vi "Synchros Final.vi"() -> ()   [LabVIEW 2014]
panel:
  out "x >= y?":bool
  in  "Tab Control":T1(tab)
  out "?":i32
  in  "?":dbl(knob) scale=0.0..360.0
  out "?":dbl(knob) scale=0.0..360.0
  out "?":dbl(knob) scale=0.0..360.0
  out "?":dbl(knob) scale=0.0..360.0
  out "?":i32
  in  "?":enum16{"S1 and S2", "S2 and S3", "S1 and S3"}(ring)
  out "?":dbl format="%#_4g"
  out "?":bool
  out "?":bool
  in  "STOP":bool
  in  "STOP  .":bool
  out "1":string[][](table)
  in  "?":dbl(slide)=29.292929292929294 scale=0.0..100.0
  out "?":dbl
  out "?":dbl(knob) scale=0.0..360.0
  out "?":dbl(knob) scale=0.0..360.0
  out "?":dbl(knob) scale=0.0..360.0
  out "?":dbl
  out "?":dbl
  in  "?":enum16{"S1 and S2", "S2 and S3", "S1 and S3"}(ring)
  out "?":dbl format="%#_4g"
  out "?":dbl(knob) scale=0.0..360.0
  out "Position Vs Stator Voltage":cluster{"Y":dbl[], "Y":dbl[]}[](graph)
  out "?":bool
  out "?":bool
  # "Manipal Institute of Technology  \n        Dept of Instrumentation and Control Engineering\n                                 V Sem (Instrumentation Lab)"
  # "VIRTUAL LABS"
  # "VIRTUAL LABS"
  # "Characteristics of Synchros\nAim:\nTo measure the Stator output voltage with respect to rotor position and plot the graph. \nApparatus required:\n1.\tSynchro Transmitter / Receiver (PEC 03) Trainer kit.\n2.\tPatch chords\n\nInstructions:\n\tConnect Digital Voltmeter across any two Stator output of Synchro transmitter.\n1.\tConnect Synchro transmitter stator outputs to corresponding Stator terminals of Synchro receiver.\n2.\tPower 'ON'  all ON/OFF Switches\n3.\tVerify the Stator output voltage of 0V at 0 degree, if it is not make 0V at 0 degree to adjust the pointer of both transmitter and Receiver.\n4.\tAdjust the transmitter rotor position Step by Step.\n5.\tNote down the output voltage for various rotor position in table 1.\n6.\tNote down the rotor position of transmitter and receiver in table 2.\n7.\tRepeat the Same procedure for other pair of Synchro transmitter coils.\n\n\nMotor graph:"
  # "EXPERIMENT NO.1"
  # "Angular Displacement\n(in deg)"
  # "Angular Displacement\n(in deg)"
  # "Reciever"
  # "Transmitter"
  # "S1"
  # "S2"
  # "S3"
  # "S1"
  # "S2"
  # "S3"
  # "Select coils for Voltage  \n    Measurement"
  # "Voltage (V)"
  # "Angular Displacement\n(in deg)"
  # "Angular Displacement\n(in deg)"
  # "Animation Speed"
  # "Reciever"
  # "Transmitter"
  # "S1"
  # "S2"
  # "S3"
  # "S1"
  # "S2"
  # "S3"
  # "Select coils for Voltage  \n    Measurement"
  # "Voltage (V)"
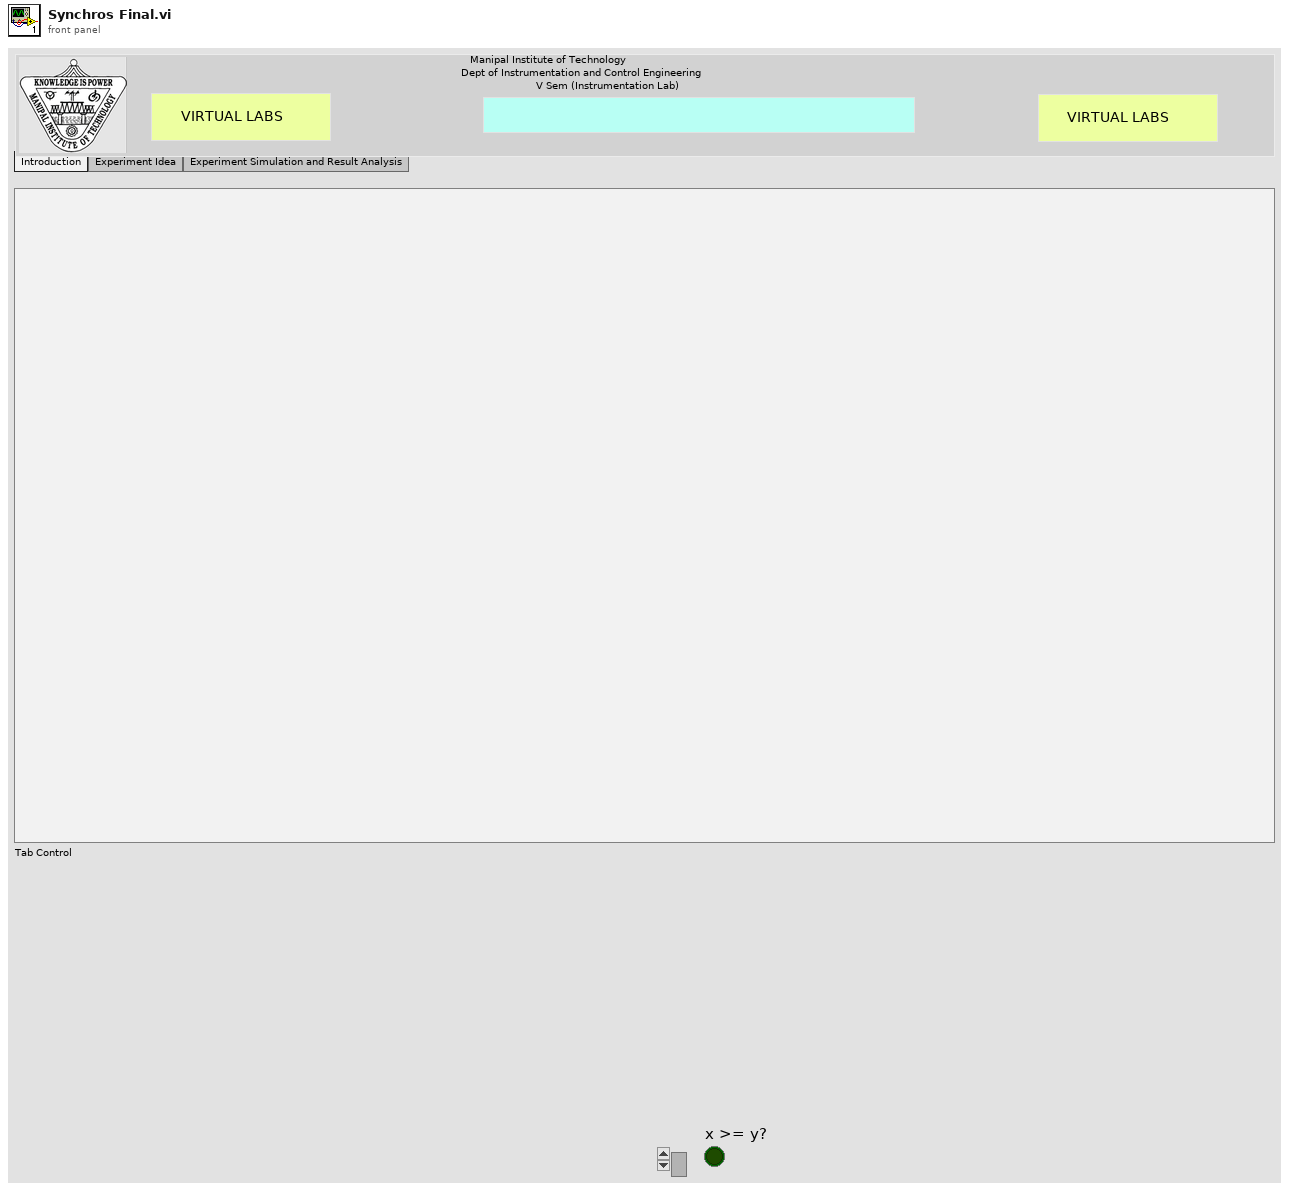
[diagram p1: front panel]
types:
  T1 = enum32{"Introduction", "Experiment Idea", "Experiment Simulation and Result Analysis"}
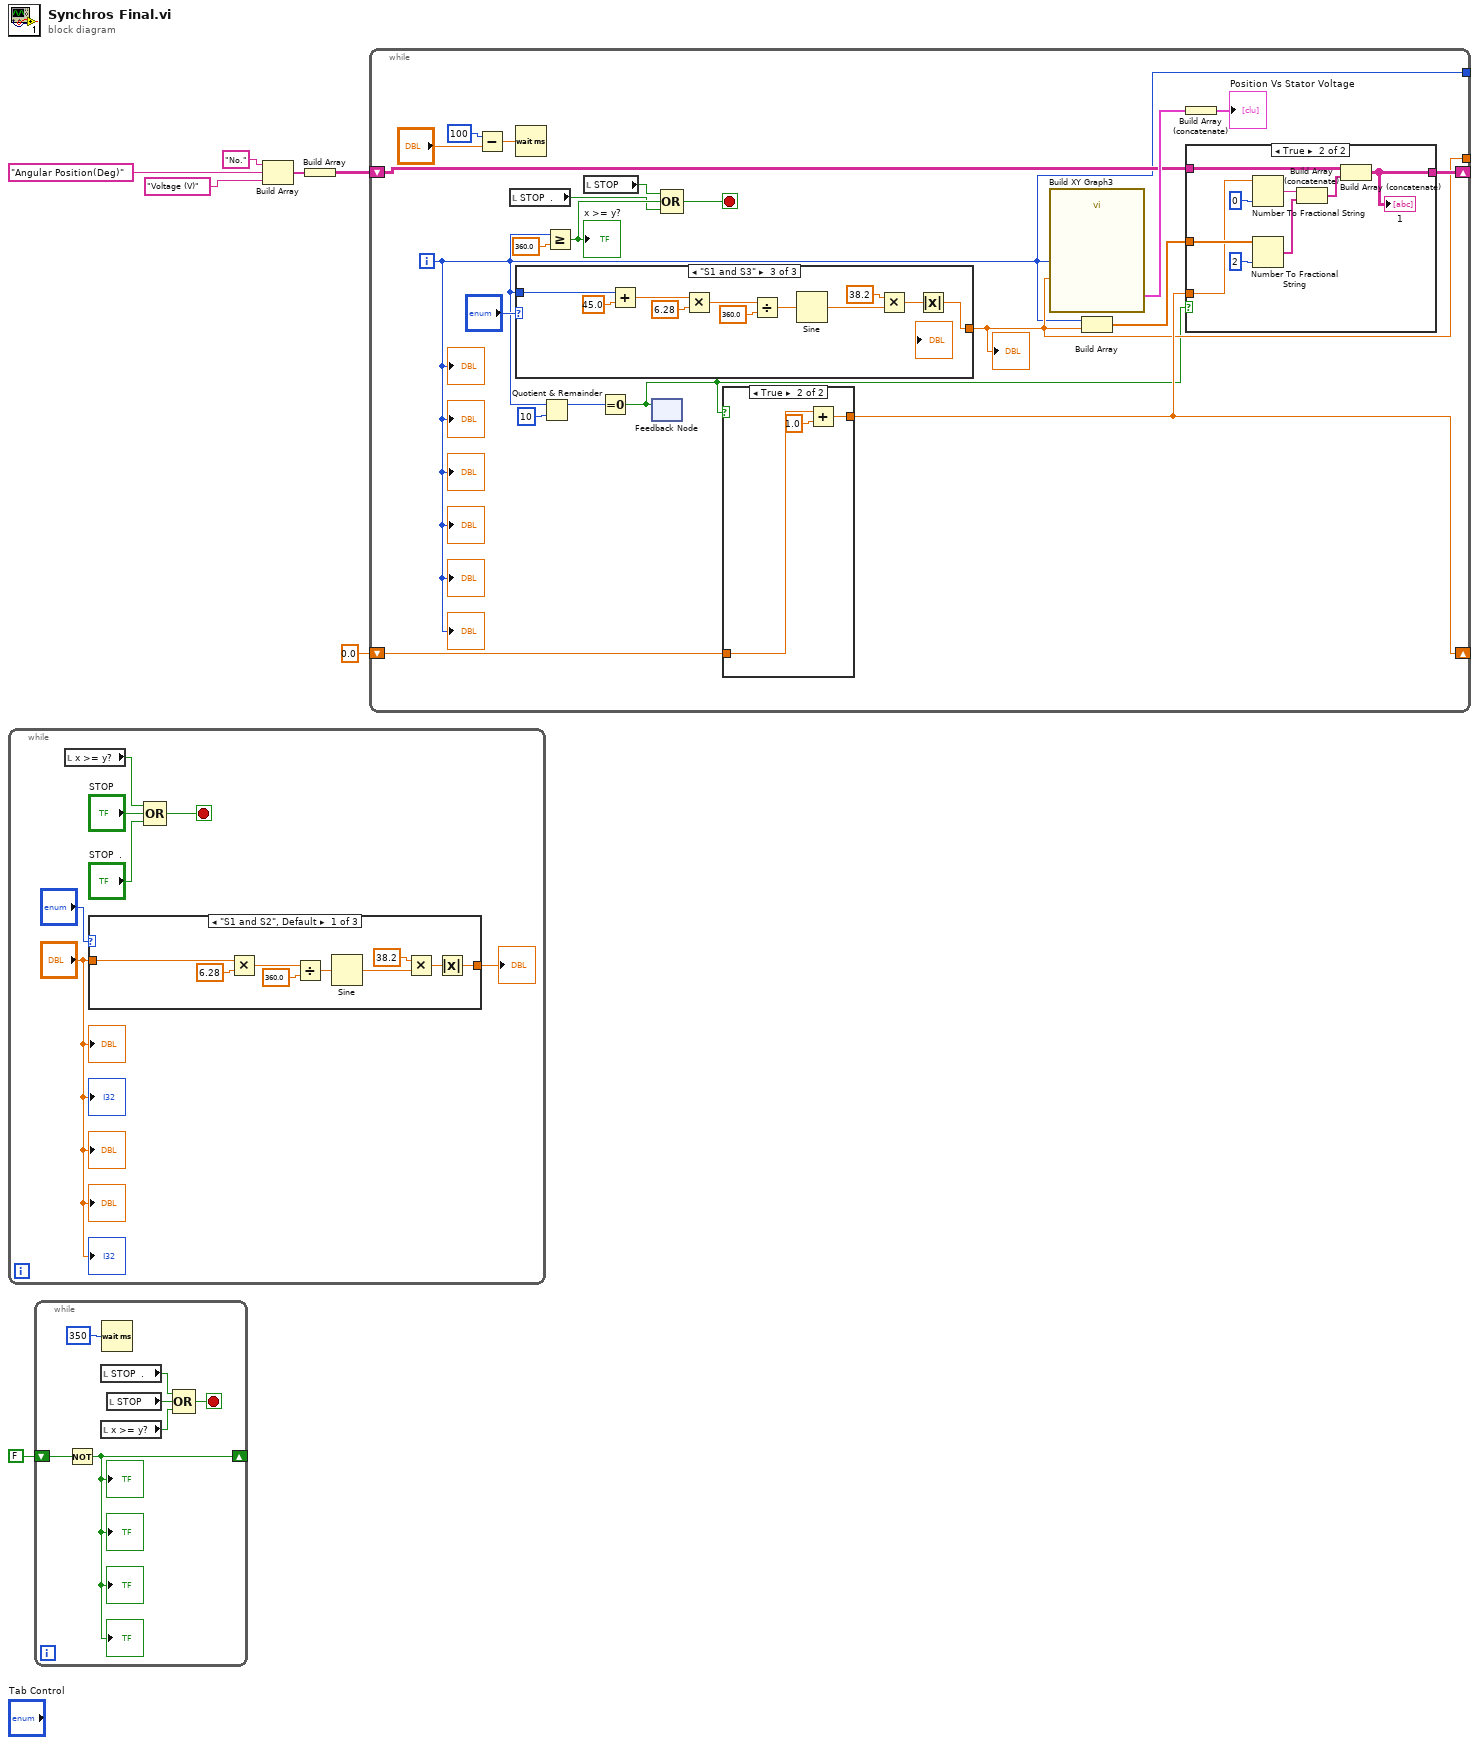
[diagram p0: block diagram]
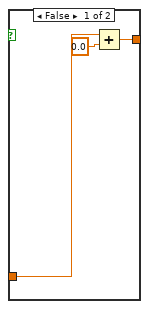
[diagram p2: hidden frame]
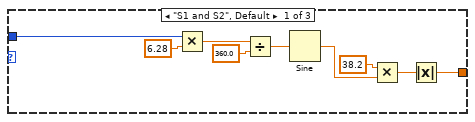
[diagram p4: hidden frame]
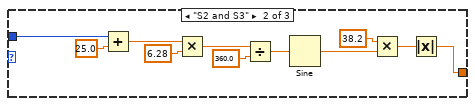
[diagram p5: hidden frame]
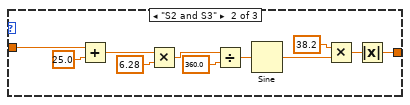
[diagram p6: hidden frame]
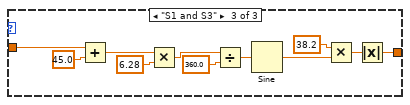
[diagram p7: hidden frame]
diagram:
  n1 = while {
    stop <- w8 stop-if-true
    n2 = local read "x >= y?"() -> (w9:bool)
    n3 = case shown="\"S1 and S2\", Default" "?" {
      tunnel: "?" -> [w16 w25 w36]
      tunnel: [w15 w24 w35] -> w13
      frame "S1 and S2", Default {
        n4 = Multiply(x=w16, y=6.28) -> (x*y=w19:dbl)
        n5 = Divide(x=w19, y=360.0) -> (x/y=w21:dbl)
        n6 = Sine(x=w21) -> (sin(x)=w22:dbl)
        n7 = Multiply(x=38.2, y=w22) -> (x*y=w23:dbl)
        n8 = Absolute Value(x=w23) -> (abs(x)=w15:dbl)
      }
      frame "S2 and S3" {
        n9 = Add(x=w25, y=25.0) -> (x+y=w34:dbl)
        n10 = Multiply(x=w34, y=6.28) -> (x*y=w30:dbl)
        n11 = Divide(x=w30, y=360.0) -> (x/y=w28:dbl)
        n12 = Sine(x=w28) -> (sin(x)=w27:dbl)
        n13 = Multiply(x=38.2, y=w27) -> (x*y=w26:dbl)
        n14 = Absolute Value(x=w26) -> (abs(x)=w24:dbl)
      }
      frame "S1 and S3" {
        n15 = Add(x=w36, y=45.0) -> (x+y=w37:dbl)
        n16 = Multiply(x=w37, y=6.28) -> (x*y=w41:dbl)
        n17 = Divide(x=w41, y=360.0) -> (x/y=w43:dbl)
        n18 = Sine(x=w43) -> (sin(x)=w44:dbl)
        n19 = Multiply(x=38.2, y=w44) -> (x*y=w45:dbl)
        n20 = Absolute Value(x=w45) -> (abs(x)=w35:dbl)
      }
    }
    "?" <- w13
    n21 = Compound Arithmetic op=OR(w9, "STOP", "STOP  .") -> (w8:bool)
    "?" <- "?"
    "?" <- "?"
    "?" <- "?"
    "?" <- "?"
    "?" <- "?"
  }
  n22 = while {
    shift-right: [w50] -> _
    shift-left: FALSE -> [w52]
    stop <- w46 stop-if-true
    n23 = Not(x=w52) -> (.not. x?=w50:bool)
    "?" <- w50
    "?" <- w50
    "?" <- w50
    "?" <- w50
    n24 = local read "STOP  ."() -> (w49:bool)
    n25 = local read "x >= y?"() -> (w47:bool)
    n26 = Wait (ms)(milliseconds to wait=u32 350) -> ()  [unwired: 1 out]
    n27 = local read "STOP"() -> (w48:bool)
    n28 = Compound Arithmetic op=OR(w49, w48, w47) -> (w46:bool)
  }
  n29 = Build Array("No." ("element"), "Angular Position(Deg)" ("element"), "Voltage (V)") -> (w4:string[])
  n30 = Build Array(w4) -> (w3:string[][])
  n31 = while {
    tunnel: [w59] -> _
    tunnel: [w57] -> _
    shift-right: [w65] -> _
    shift-left: w3 -> [w66]
    shift-right: [w60] -> _
    shift-left: 0.0 -> [w62]
    i -> [w57]
    stop <- w54 stop-if-true
    n32 = Subtract(x=u32 100 ("milliseconds to wait"), y="?") -> (x-y=w68:dbl)
    n33 = local read "STOP  ."() -> (w53:bool)
    n34 = Wait (ms)(milliseconds to wait=w68) -> ()  [unwired: 1 out]
    n35 = case shown="\"S1 and S3\"" "?" {
      tunnel: w57 -> [w91 w100 w111]
      tunnel: [w90 w99 w110] -> w59
      frame "S1 and S2", Default {
        n36 = Multiply(x=w91, y=6.28) -> (x*y=w94:dbl)
        n37 = Divide(x=w94, y=360.0) -> (x/y=w96:dbl)
        n38 = Sine(x=w96) -> (sin(x)=w97:dbl)
        n39 = Multiply(x=38.2, y=w97) -> (x*y=w98:dbl)
        n40 = Absolute Value(x=w98) -> (abs(x)=w90:dbl)
      }
      frame "S2 and S3" {
        n41 = Add(x=w100, y=25.0) -> (x+y=w109:dbl)
        n42 = Multiply(x=w109, y=6.28) -> (x*y=w105:dbl)
        n43 = Divide(x=w105, y=360.0) -> (x/y=w103:dbl)
        n44 = Sine(x=w103) -> (sin(x)=w102:dbl)
        n45 = Multiply(x=38.2, y=w102) -> (x*y=w101:dbl)
        n46 = Absolute Value(x=w101) -> (abs(x)=w99:dbl)
      }
      frame "S1 and S3" {
        n47 = Add(x=w111, y=45.0) -> (x+y=w112:dbl)
        n48 = Multiply(x=w112, y=6.28) -> (x*y=w116:dbl)
        n49 = Divide(x=w116, y=360.0) -> (x/y=w118:dbl)
        n50 = Sine(x=w118) -> (sin(x)=w119:dbl)
        n51 = Multiply(x=38.2, y=w119) -> (x*y=w120:dbl)
        n52 = Absolute Value(x=w120) -> (abs(x)=w110:dbl)
      }
    }
    "?" <- w59
    n53 = Quotient & Remainder(x=w57, y=10) -> (x-y*floor(x/y)=w64:i32)  [unwired: 1 out]
    n54 = Greater Or Equal?(x=w57, y=360.0) -> (x >= y?=w56:bool)
    "x >= y?" <- w56
    n55 = local read "STOP"() -> (w55:bool)
    n56 = Equal To 0?(x=w64) -> (x = 0?=w58:bool)
    n57 = feedback-in #1(w58) -> ()
    n58 = feedback #1() -> ()  [unwired: 2 in]
    n59 = Compound Arithmetic op=OR(w55, w56, w53) -> (w54:bool)
    n60 = case shown="True" w58 {
      tunnel: w62 -> [w75 w79]
      tunnel: [w74 w78] -> w60
      frame False {
        n61 = Add(x=w75, y=0.0) -> (x+y=w74:dbl)
      }
      frame True {
        n62 = Add(x=w79, y=1.0) -> (x+y=w78:dbl)
      }
    }
    n63 = call "Build XY Graph3"("Y Input"=w59, "X Input"=w57) -> ("XY Graph"=w70:cluster{"Y":dbl[], "Y":dbl[]}[])  [unwired: 3 in, 6 out]
    n64 = Build Array(w57, w59) -> (w61:dbl[])
    n65 = Build Array (concatenate)(w70) -> (→"Position Vs Stator Voltage":cluster{"Y":dbl[], "Y":dbl[]}[])
    n66 = case shown="True" w58 {
      tunnel: w61 -> [_ w89]
      tunnel: w66 -> [w80 w82]
      tunnel: [w80 w81] -> w65
      tunnel: w60 -> [_ w87]
      frame False {
      }
      frame True {
        n67 = Number To Fractional String(number=w87, precision (6)=i16 0) -> (F-format string=w85:string)  [unwired: 2 in]
        n68 = Number To Fractional String(number=w89, precision (6)=i16 2) -> (F-format string=w84:string[])  [unwired: 2 in]
        n69 = Build Array (concatenate)(w85, w84) -> (w83:string[])
        n70 = Build Array (concatenate)(w82, w83) -> (w81:string[][])
        "1" <- w81
      }
    }
    "?" <- w57
    "?" <- w57
    "?" <- w57
    "?" <- w57
    "?" <- w57
    "?" <- w57
  }
